vi "pattern_tag.vi"(1 "U":ext[][](array[numeric])) -> (0 "tag":i32[](array[numeric]))   [LabVIEW 2009]
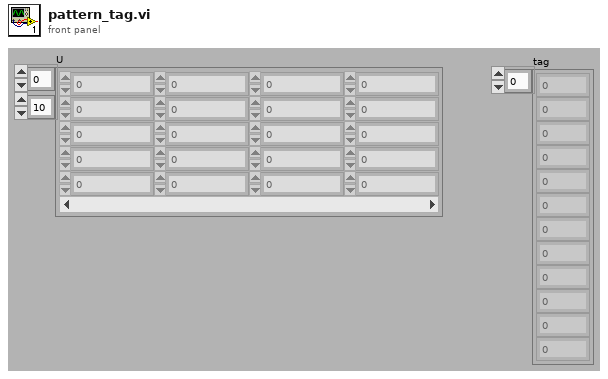
[diagram p1: front panel]
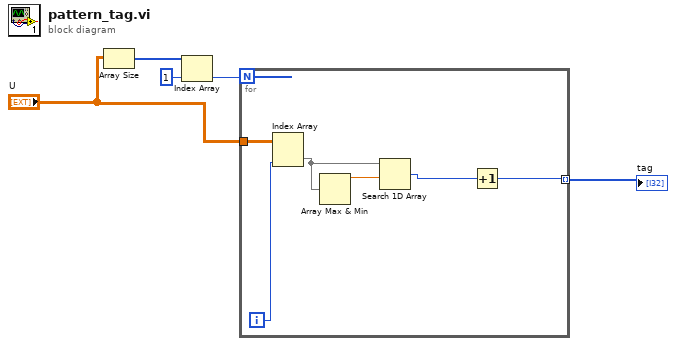
[diagram p0: block diagram]
diagram:
  n1 = Array Size(array="U") -> (size(s)=w5:i32[])
  n2 = Index Array(array=w5, index=1) -> (element=w3:i32)
  n3 = for {
    N: w3 -> [_]
    tunnel: "U" -> [w11]
    tunnel: [w6] -> w2 mode=indexing
    i -> [w10]
    n4 = Index Array(array=w11, index (col)=w10) -> (element=w9:ext[])  [unwired: 1 in]
    n5 = Array Max & Min(array=w9) -> (max value=w8:ext)  [unwired: 3 out]
    n6 = Search 1D Array(1D array=w9, element=w8) -> (index of element=w7:i32)  [unwired: 1 in]
    n7 = Increment(x=w7) -> (x+1=w6:i32)
  }
  "tag" <- w2
